vi "experiment control.vi"() -> ()   [LabVIEW 2012] (continued)
            n2214 = Decimal String To Number(string=w4963) -> (number=w4964:i32)  [unwired: 2 in, 1 out]
            n2215 = local read "DAC Schedule"() -> (w4965:T6)
            n2216 = local read "DAC Tasks"() -> (w4966:T8)
            n2217 = call "DAC compile.vi"("DAC Tasks"=w4966, "DAC Schedule"=w4965, "index"=w4964) -> ("DAC"=w4962:cluster{"Time":dbl, "Voltage":dbl[]}[])  [unwired: 8 in]
            n2218 = for {
              tunnel: w4962 -> [w4976] mode=indexing
              tunnel: [w4975] -> w4961 mode=indexing
              tunnel: [w4974] -> w4958 mode=indexing
              n2219 = Unbundle By Name(w4976) -> ("Time"=w4975:dbl, "Voltage"=w4974:dbl[])
            }
            n2220 = Transpose 2D Array(2D array=w4958) -> (transposed array=w4959:dbl[][])
            n2221 = for {
              tunnel: w4959 -> [w4972] mode=indexing
              tunnel: w4961 -> [w4973]
              tunnel: [w4971] -> w4960 mode=indexing
              n2222 = Bundle(w4973, w4972) -> (w4971:cluster{dbl[], dbl[]})  [unwired: 1 in]
            }
            "DAC View" <- w4960
          }
          frame "DAC: Clear" {
            n2223 = Unbundle By Name(w4982) -> ("dac state"=w4984:T7)
            n2224 = Unbundle By Name(w4984) -> ("loaded"=w4985:bool)
            n2225 = call <vilib>:"Clear Errors.vi"("error in (no error)"=w4978) -> ("error out"=w4980:errorcluster)  [unwired: 6 in]
            n2226 = case shown="True" w4985 {
              tunnel: [w4991 w5000] -> w4979
              tunnel: w4980 -> [w4994 w5000]
              tunnel: w4984 -> [w4988 w4999]
              tunnel: [w4987 w4999] -> w4983
              frame True {
                n2227 = Unbundle By Name(w4988) -> ("output 1"=w4998:refnum<k21>, "clock 1"=w4997:refnum<k21>, "output 2"=w4989:refnum<k21>, "clock 2"=w4990:refnum<k21>)
                n2228 = call <vilib>:"DAQmx Clear Task.vi"("task in"=w4998, "error in"=w4994) -> ("error out"=w4995:errorcluster)  [unwired: 13 in]
                n2229 = call <vilib>:"DAQmx Clear Task.vi"("task in"=w4997, "error in"=w4995) -> ("error out"=w4992:errorcluster)  [unwired: 13 in]
                n2230 = call <vilib>:"DAQmx Clear Task.vi"("task in"=w4989, "error in"=w4992) -> ("error out"=w4993:errorcluster)  [unwired: 13 in]
                n2231 = Bundle By Name(cluster=w4988, "loaded"=FALSE) -> (w4987:T7)
                n2232 = call <vilib>:"DAQmx Clear Task.vi"("task in"=w4990, "error in"=w4993) -> ("error out"=w4991:errorcluster)  [unwired: 13 in]
              }
              frame False {
              }
            }
            n2233 = Merge Errors(w4979, w4978) -> (w4977:errorcluster)
            n2234 = Bundle By Name(cluster=w4982, "dac state"=w4983) -> (w4981:T52)
          }
          frame "----------- Depletion Agilent -----------" {
            # "Template Separator\n(You can make a copy of, or modify, this frame)"
          }
          frame "Depletion Agilent: Initialize" {
            w5004 = TRUE ("Enable Output  (T: Enable)")
            # "Use this as a template for any command that you might want to profile."
            n2235 = local read "Depletion Agilent"() -> (w5006:T14)
            n2236 = Unbundle By Name(w5006) -> ("USB"=w5010:refnum<visa-resource-name>)
            n2237 = call <instrlib>:"Initialize.vi"("Serial Configuration"=T50 {"Baud Rate"=9600, "Parity"=0, "Data Bits"=8, "Flow Control"=4}, "error in (no error)"=w5013, "VISA resource name"=w5010) -> ("error out"=w5008:errorcluster, "VISA resource name out"=w5007:refnum<visa-resource-name>)  [unwired: 7 in]
            n2238 = call <instrlib>:"Enable Output.vi"("error in (no error)"=w5008, "Enable Output  (T: Enable)"=w5004, "VISA resource name"=w5007) -> ("error out"=w5012:errorcluster)  [unwired: 7 in, 1 out]
            n2239 = Bundle By Name(cluster=w5006, "Output"=w5004) -> (w5005:T14)
            n2240 = local write "Depletion Agilent"(w5005) -> ()
          }
          frame "Depletion Agilent: Set" {
            w5043 = u16 0 items=["50 Ohms", "High Impedance", "User Defined"] ("Impedance (0: 50 Ohms)")
            # "Use this as a template for any command that you might want to profile."
            n2241 = local read "Depletion Agilent"() -> (w5016:T14)
            n2242 = Unbundle By Name(w5016) -> ("Channels"=w5023:T96, "Output Select"=w5024:bool, "Amplitude"=w5020:dbl, "Offset"=w5019:dbl, "USB"=w5025:refnum<visa-resource-name>)
            n2243 = Boolean To (0,1)(Boolean=w5024) -> (0, 1=w5042:i16)
            n2244 = Delete From Array(array=w5023, index=w5042) -> (deleted portion=w5041:T97)  [unwired: 1 in, 1 out]
            n2245 = Unbundle By Name(w5041) -> ("Trigger"=w5018:bool, "Phase"=w5017:dbl, "Frequency"=w5022:dbl, "Duty Cycle"=w5021:dbl)
            n2246 = call <instrlib>:"Configure Output Impedance.vi"("error in (no error)"=w5045, "Impedance (0: 50 Ohms)"=w5043, "VISA resource name"=w5025) -> ("error out"=w5031:errorcluster, "VISA resource name out"=w5029:refnum<visa-resource-name>)  [unwired: 7 in]
            n2247 = Boolean To (0,1)(Boolean=w5018) -> (0, 1=w5035:i16)
            n2248 = Format Into String(format string="%.;:FREQ %f;:VOLT %g;:VOLT:OFFS %g;:FUNC:SQU:DCYC %f" ("Frequency Command"), initial string="FUNC:SHAP SQU;:VOLT:UNIT VPP;" ("string (\"\")"), w5022, w5020, w5019, w5021) -> (resulting string=w5034:string)  [unwired: 1 in, 1 out]
            n2249 = VISA Write(VISA resource name=w5029, write buffer=w5034, error in (no error)=w5031) -> (VISA resource name out=w5028:refnum<visa-resource-name>, error out=w5030:errorcluster)  [unwired: 1 out]
            n2250 = Pick Line(multi-line string="BURS:MODE TRIG;\nBURS:MODE GAT;" ("f"), line index=w5035) -> (output string=w5038:string)  [unwired: 1 in]
            n2251 = Format Into String(format string="%.;:BURS:PHAS %f;", initial string=w5038, w5017) -> (resulting string=w5027:string)  [unwired: 1 in, 1 out]
            n2252 = case shown="True" w5018 {
              tunnel: w5027 -> [w5049 w5052]
              tunnel: [w5047 w5050] -> w5026
              frame False {
                n2253 = Concatenate Strings(w5049, ":BURS:NCYC 10;:TRIG:SOUR IMM;") -> (w5047:string)
              }
              frame True {
                n2254 = Concatenate Strings(w5052, ":TRIG:SOUR EXT;:BURS:NCYC INF;") -> (w5050:string)
              }
            }
            n2255 = Concatenate Strings(w5026, ":BURS:STAT ON;") -> (w5032:string)
            n2256 = VISA Write(VISA resource name=w5028, write buffer=w5032, error in (no error)=w5030) -> (error out=w5015:errorcluster)  [unwired: 2 out]
          }
          frame "Depletion Agilent: Output" {
            # "Use this as a template for any command that you might want to profile."
            n2257 = local read "Depletion Agilent"() -> (w5055:T14)
            n2258 = Unbundle By Name(w5055) -> ("USB"=w5054:refnum<visa-resource-name>, "Output"=w5053:bool)
            n2259 = call <instrlib>:"Enable Output.vi"("error in (no error)"=w5058, "Enable Output  (T: Enable)"=w5053, "VISA resource name"=w5054) -> ("error out"=w5057:errorcluster)  [unwired: 7 in, 1 out]
          }
          frame "Depletion Agilent: Close" {
            # "Use this as a template for any command that you might want to profile."
            n2260 = local read "Depletion Agilent"() -> (w5062:T14)
            n2261 = Unbundle By Name(w5062) -> ("USB"=w5061:refnum<visa-resource-name>)
            n2262 = call <instrlib>:"Close.vi"("error in (no error)"=w5064, "VISA resource name"=w5061) -> ("error out"=w5063:errorcluster)  [unwired: 9 in]
          }
          frame "-----------Chillax-----------" {
            # "Template Separator\n(You can make a copy of, or modify, this frame)"
          }
          frame "Chillax: Initialize" {
            # "Use this as a template for any command that you might want to profile."
            n2263 = local read "Chillax"() -> (w5104:T12)
            n2264 = Unbundle By Name(w5104) -> ("Chillax Voltage"=w5097:dbl, "Chillax"=w5107:refnum<visa-resource-name>, "Output"=w5069:bool)
            n2265 = call <instrlib>:"Initialize.vi"("error in (no error)"=w5109, "VISA resource name"=w5107) -> ("error out"=w5106:errorcluster, "VISA resource name out"=w5105:refnum<visa-resource-name>)  [unwired: 8 in]
            n2266 = local read "Chillax"() -> (w5100:T12)
            n2267 = call <instrlib>:"Enable Output.vi"("error in (no error)"=w5106, "Enable Output  (T: Enable)"=w5069, "VISA resource name"=w5105) -> ("error out"=w5102:errorcluster, "VISA resource name out"=w5103:refnum<visa-resource-name>)  [unwired: 7 in]
            n2268 = Bundle By Name(cluster=w5100, "Output"=w5069) -> (w5099:T12)
            n2269 = Negate(x=w5097) -> (-x=w5096:dbl)
            n2270 = call "ag33xxx - Select User Def Wfm.vi"("error in (no error)"=w5102, "User Def. Wfm Name"="CHILLAX", "VISA session"=w5103) -> ("error out"=w5091:errorcluster, "dup VISA session"=w5092:refnum<visa-resource-name>)  [unwired: 7 in]
            n2271 = Format Into String(format string=":VOLT:HIGH 0;:VOLT:LOW %g;", w5096) -> (resulting string=w5090:string)  [unwired: 2 in, 1 out]
            n2272 = local write "Chillax"(w5099) -> ()
            n2273 = Format Into String(format string=":BURS:STAT ON;:BURS:MODE TRIG;:BURS:NCYC 1;:BURS:PHAS 0;:TRIG:SOUR EXT;:PULS:PER %g;", initial string=w5090, 0.013 ("input 1")) -> (resulting string=w5094:string)  [unwired: 1 in, 1 out]
            n2274 = VISA Write(VISA resource name=w5092, write buffer=w5094, error in (no error)=w5091) -> (error out=w5074:errorcluster)  [unwired: 2 out]
            n2275 = local read "Chillax"() -> (w5075:T12)
            n2276 = Unbundle By Name(w5075) -> ("Chillax Voltage"=w5071:dbl, "Unchillax"=w5072:refnum<visa-resource-name>, "Output"=w5070:bool)
            n2277 = call <instrlib>:"Initialize.vi"("error in (no error)"=w5074, "VISA resource name"=w5072) -> ("error out"=w5076:errorcluster, "VISA resource name out"=w5077:refnum<visa-resource-name>)  [unwired: 8 in]
            n2278 = local read "Chillax"() -> (w5081:T12)
            n2279 = call <instrlib>:"Enable Output.vi"("error in (no error)"=w5076, "Enable Output  (T: Enable)"=w5070, "VISA resource name"=w5077) -> ("error out"=w5079:errorcluster, "VISA resource name out"=w5078:refnum<visa-resource-name>)  [unwired: 7 in]
            n2280 = Bundle By Name(cluster=w5081, "Output"=w5070) -> (w5082:T12)
            n2281 = call "ag33xxx - Select User Def Wfm.vi"("error in (no error)"=w5079, "User Def. Wfm Name"="UNCHILLAX", "VISA session"=w5078) -> ("error out"=w5088:errorcluster, "dup VISA session"=w5087:refnum<visa-resource-name>)  [unwired: 7 in]
            n2282 = Format Into String(format string=":VOLT:LOW 0;:VOLT:HIGH %g;", w5071) -> (resulting string=w5089:string)  [unwired: 2 in, 1 out]
            n2283 = local write "Chillax"(w5082) -> ()
            n2284 = Format Into String(format string=":BURS:STAT ON;:BURS:MODE TRIG;:BURS:NCYC 1;:BURS:PHAS 0;:TRIG:SOUR EXT;:PULS:PER %g;", initial string=w5089, 0.13 ("input 1")) -> (resulting string=w5085:string)  [unwired: 1 in, 1 out]
            n2285 = VISA Write(VISA resource name=w5087, write buffer=w5085, error in (no error)=w5088) -> (error out=w5073:errorcluster)  [unwired: 2 out]
          }
          frame "Chillax: Close" {
            # "Use this as a template for any command that you might want to profile."
            n2286 = local read "Chillax"() -> (w5116:T12)
            n2287 = Unbundle By Name(w5116) -> ("Unchillax"=w5113:refnum<visa-resource-name>, "Chillax"=w5115:refnum<visa-resource-name>)
            n2288 = call "ag33xxx - Close.vi"("error in (no error)"=w5114, "VISA session"=w5115) -> ("error out"=w5112:errorcluster)  [unwired: 9 in]
            n2289 = call "ag33xxx - Close.vi"("error in (no error)"=w5112, "VISA session"=w5113) -> ("error out"=w5111:errorcluster)  [unwired: 9 in]
          }
          frame "Chillax: Set Voltage" {
            # "Use this as a template for any command that you might want to profile."
            n2290 = local read "Chillax"() -> (w5130:T12)
            n2291 = Unbundle By Name(w5130) -> ("Chillax Voltage"=w5120:dbl, "Chillax"=w5127:refnum<visa-resource-name>, "Unchillax"=w5119:refnum<visa-resource-name>)
            n2292 = Negate(x=w5120) -> (-x=w5121:dbl)
            n2293 = Format Into String(format string=":VOLT:HIGH 0;:VOLT:LOW %g;" ("Amplitude Command"), w5121) -> (resulting string=w5126:string)  [unwired: 2 in, 1 out]
            n2294 = VISA Write(VISA resource name=w5127, write buffer=w5126, error in (no error)=w5129) -> (error out=w5124:errorcluster)  [unwired: 2 out]
            n2295 = Format Into String(format string=":VOLT:LOW 0;:VOLT:HIGH %g;" ("Amplitude Command"), w5120) -> (resulting string=w5125:string)  [unwired: 2 in, 1 out]
            n2296 = VISA Write(VISA resource name=w5119, write buffer=w5125, error in (no error)=w5124) -> (error out=w5123:errorcluster)  [unwired: 2 out]
          }
          frame "Chillax: Output" {
            # "Use this as a template for any command that you might want to profile."
            n2297 = local read "Chillax"() -> (w5139:T12)
            n2298 = Unbundle By Name(w5139) -> ("Unchillax"=w5136:refnum<visa-resource-name>, "Chillax"=w5138:refnum<visa-resource-name>, "Output"=w5133:bool)
            n2299 = call <instrlib>:"Enable Output.vi"("error in (no error)"=w5137, "Enable Output  (T: Enable)"=w5133, "VISA resource name"=w5138) -> ("error out"=w5135:errorcluster)  [unwired: 7 in, 1 out]
            n2300 = call <instrlib>:"Enable Output.vi"("error in (no error)"=w5135, "Enable Output  (T: Enable)"=w5133, "VISA resource name"=w5136) -> ("error out"=w5134:errorcluster)  [unwired: 7 in, 1 out]
          }
          frame "----------- Trap Agilent -----------" {
            # "Template Separator\n(You can make a copy of, or modify, this frame)"
          }
          frame "Trap Agilent: Initialize" {
            w5145 = TRUE ("Enable Output  (T: Enable)")
            # "Use this as a template for any command that you might want to profile."
            n2301 = local read "Trap Agilent"() -> (w5147:T13)
            n2302 = Unbundle By Name(w5147) -> ("USB"=w5151:refnum<visa-resource-name>)
            n2303 = call <instrlib>:"Initialize.vi"("Serial Configuration"=T50 {"Baud Rate"=9600, "Parity"=0, "Data Bits"=8, "Flow Control"=4}, "error in (no error)"=w5154, "VISA resource name"=w5151) -> ("error out"=w5149:errorcluster, "VISA resource name out"=w5148:refnum<visa-resource-name>)  [unwired: 7 in]
            n2304 = call <instrlib>:"Enable Output.vi"("error in (no error)"=w5149, "Enable Output  (T: Enable)"=w5145, "VISA resource name"=w5148) -> ("error out"=w5153:errorcluster)  [unwired: 7 in, 1 out]
            n2305 = Bundle By Name(cluster=w5147, "Output"=w5145) -> (w5146:T13)
            n2306 = local write "Trap Agilent"(w5146) -> ()
          }
          frame "Trap Agilent: Set" {
            w5157 = u16 1 items=["DC", "Sine", "Square", "Triangle", "Ramp", "Pulse", "Noise", "Sinc", "Negative Ramp", "Exponential Rise", "Exponential Fall", "Cardiac"] ("Waveform Function (1: Sine)")
            w5163 = u16 0 items=["Vpp", "Vrms", "dB"] ("Unit (0: Vpp)")
            w5166 = u16 1 items=["50 Ohms", "High Impedance", "User Defined"] ("Impedance (0: 50 Ohms)")
            w5169 = u16 1 items=["Triggered", "Gated"] ("Burst Mode (0: Triggered)")
            # "Use this as a template for any command that you might want to profile."
            n2307 = local read "Trap Agilent"() -> (w5172:T13)
            n2308 = Unbundle By Name(w5172) -> ("Phase"=w5171:dbl, "Frequency"=w5173:dbl, "USB"=w5156:refnum<visa-resource-name>, "Amplitude"=w5164:dbl)
            n2309 = Divide(x=w5164, y=1000.0) -> (x/y=w5160:dbl)
            n2310 = Multiply(x=1000.0, y=w5173) -> (x*y=w5159:dbl)
            n2311 = call <instrlib>:"Configure Burst.vi"("Burst Mode (0: Triggered)"=w5169, "error in (no error)"=w5177, "Burst Phase (0 deg)"=w5171, "Enable Burst (T: Enable)"=TRUE, "VISA resource name"=w5156) -> ("error out"=w5168:errorcluster, "VISA resource name out"=w5167:refnum<visa-resource-name>)  [unwired: 5 in]
            n2312 = call <instrlib>:"Configure Output Impedance.vi"("error in (no error)"=w5168, "Impedance (0: 50 Ohms)"=w5166, "VISA resource name"=w5167) -> ("error out"=w5161:errorcluster, "VISA resource name out"=w5162:refnum<visa-resource-name>)  [unwired: 7 in]
            n2313 = call <instrlib>:"Configure Standard Waveform.vi"("Unit (0: Vpp)"=w5163, "DC Offset (0.00 V)"=0.0, "Frequency (1000 Hz)"=w5159, "error in (no error)"=w5161, "Amplitude (1)"=w5160, "Waveform Function (1: Sine)"=w5157, "VISA resource name"=w5162) -> ("error out"=w5176:errorcluster)  [unwired: 3 in, 1 out]
          }
          frame "Trap Agilent: Output" {
            # "Use this as a template for any command that you might want to profile."
            n2314 = local read "Trap Agilent"() -> (w5181:T13)
            n2315 = Unbundle By Name(w5181) -> ("USB"=w5180:refnum<visa-resource-name>, "Output"=w5179:bool)
            n2316 = call <instrlib>:"Enable Output.vi"("error in (no error)"=w5184, "Enable Output  (T: Enable)"=w5179, "VISA resource name"=w5180) -> ("error out"=w5183:errorcluster)  [unwired: 7 in, 1 out]
          }
          frame "Trap Agilent: Close" {
            # "Use this as a template for any command that you might want to profile."
            n2317 = local read "Trap Agilent"() -> (w5188:T13)
            n2318 = Unbundle By Name(w5188) -> ("USB"=w5187:refnum<visa-resource-name>)
            n2319 = call <instrlib>:"Close.vi"("error in (no error)"=w5190, "VISA resource name"=w5187) -> ("error out"=w5189:errorcluster)  [unwired: 9 in]
          }
          frame "----------- USB DAQ -----------" {
            # "Template Separator\n(You can make a copy of, or modify, this frame)"
          }
          frame "USB DAQ: Initialize" {
            # "Use this as a template for any command that you might want to profile."
            n2320 = local read "USB DAQ"() -> (w5208:T11)
            n2321 = Unbundle By Name(w5208) -> ("Analog Out"=w5202:u8[], "Digital Out"=w5197:bool[])
            n2322 = dll-call lib="C:/Users/edm/Desktop/experimentcontrol/trunk/subvis/USB DAQ/K8055D.dll" fn="OpenDevice"(error in=w5212, 0) -> (error out=w5209:errorcluster)  [unwired: 4 in, 1 out]
            n2323 = Not(x=w5197) -> (.not. x?=w5196:bool[])
            n2324 = Boolean Array To Number(Boolean array=w5196) -> (number=w5207:u32)
            n2325 = dll-call lib="C:/Users/edm/Desktop/experimentcontrol/trunk/subvis/USB DAQ/K8055D.dll" fn="WriteAllDigital"(error in=w5209, w5207) -> (error out=w5206:errorcluster)  [unwired: 4 in, 1 out]
            n2326 = Delete From Array(array=w5202, index=0) -> (deleted portion=w5201:u8)  [unwired: 1 in, 1 out]
            n2327 = dll-call lib="C:/Users/edm/Desktop/experimentcontrol/trunk/subvis/USB DAQ/K8055D.dll" fn="OutputAnalogChannel"(error in=w5206, 1, w5201) -> (error out=w5203:errorcluster)  [unwired: 5 in, 1 out]
            n2328 = Delete From Array(array=w5202, index=1) -> (deleted portion=w5200:u8)  [unwired: 1 in, 1 out]
            n2329 = dll-call lib="C:/Users/edm/Desktop/experimentcontrol/trunk/subvis/USB DAQ/K8055D.dll" fn="OutputAnalogChannel"(error in=w5203, 2, w5200) -> (error out=w5211:errorcluster)  [unwired: 5 in, 1 out]
          }
          frame "USB DAQ: Digital Write" {
            # "Use this as a template for any command that you might want to profile."
            n2330 = local read "USB DAQ"() -> (w5222:T11)
            n2331 = Match Pattern(string=w5232, regular expression=",") -> (before substring=w5228:string, after substring=w5227:string)  [unwired: 1 in, 2 out]
            n2332 = Decimal String To Number(string=w5227) -> (number=w5226:i32)  [unwired: 2 in, 1 out]
            n2333 = Unbundle By Name(w5222) -> ("Digital Out"=w5221:bool[])
            n2334 = Decimal String To Number(string=w5228) -> (number=w5225:i32)  [unwired: 2 in, 1 out]
            n2335 = Number To Boolean Array(number=w5226) -> (Boolean array=w5217:bool[])
            n2336 = Decrement(x=w5225) -> (x-1=w5224:i32)
            n2337 = Not(x=w5217) -> (.not. x?=w5216:bool[])
            n2338 = Not(x=w5221) -> (.not. x?=w5220:bool[])
            n2339 = Index Array(array=w5216, index=0) -> (element=w5214:bool)
            n2340 = Replace Array Subset(array=w5220, new element=w5214, index=w5224) -> (w5219:bool[])
            n2341 = Boolean Array To Number(Boolean array=w5219) -> (number=w5230:u32)
            n2342 = dll-call lib="C:/Users/edm/Desktop/experimentcontrol/trunk/subvis/USB DAQ/K8055D.dll" fn="WriteAllDigital"(error in=w5234, w5230) -> (error out=w5233:errorcluster)  [unwired: 4 in, 1 out]
            n2343 = Not(x=w5219) -> (.not. x?=w5218:bool[])
            n2344 = Bundle By Name(cluster=w5222, "Digital Out"=w5218) -> (w5223:T11)
            n2345 = local write "USB DAQ"(w5223) -> ()
          }
          frame "USB DAQ: Digital Read" {
            # "Use this as a template for any command that you might want to profile."
            n2346 = dll-call lib="C:/Users/edm/Desktop/experimentcontrol/trunk/subvis/USB DAQ/K8055D.dll" fn="ReadAllDigital"(error in=w5243) -> (error out=w5242:errorcluster, w5240:i32)  [unwired: 2 in, 1 out]
            n2347 = Number To Boolean Array(number=w5240) -> (Boolean array=w5237:bool[])
            n2348 = local read "USB DAQ"() -> (w5239:T11)
            n2349 = Not(x=w5237) -> (.not. x?=w5236:bool[])
            n2350 = Bundle By Name(cluster=w5239, "Digital In"=w5236) -> (w5238:T11)
            n2351 = local write "USB DAQ"(w5238) -> ()
          }
          frame "USB DAQ: Analog Write" {
            # "Use this as a template for any command that you might want to profile."
            n2352 = local read "USB DAQ"() -> (w5253:T11)
            n2353 = Unbundle By Name(w5253) -> ("Analog Out"=w5245:u8[])
            n2354 = Delete From Array(array=w5245, index=0) -> (deleted portion=w5252:u8)  [unwired: 1 in, 1 out]
            n2355 = dll-call lib="C:/Users/edm/Desktop/experimentcontrol/trunk/subvis/USB DAQ/K8055D.dll" fn="OutputAnalogChannel"(error in=w5256, 1, w5252) -> (error out=w5246:errorcluster)  [unwired: 5 in, 1 out]
            n2356 = Delete From Array(array=w5245, index=1) -> (deleted portion=w5247:u8)  [unwired: 1 in, 1 out]
            n2357 = dll-call lib="C:/Users/edm/Desktop/experimentcontrol/trunk/subvis/USB DAQ/K8055D.dll" fn="OutputAnalogChannel"(error in=w5246, 2, w5247) -> (error out=w5255:errorcluster)  [unwired: 5 in, 1 out]
          }
          frame "USB DAQ: Analog Read" {
            # "Use this as a template for any command that you might want to profile."
            n2358 = dll-call lib="C:/Users/edm/Desktop/experimentcontrol/trunk/subvis/USB DAQ/K8055D.dll" fn="ReadAllAnalog"(error in=w5265) -> (error out=w5264:errorcluster, w5261:i32, w5260:i32)  [unwired: 5 in, 1 out]
            n2359 = Build Array(w5261, w5260) -> (w5259:i32[])
            n2360 = local read "USB DAQ"() -> (w5263:T11)
            n2361 = Bundle By Name(cluster=w5263, "Analog In"=w5259) -> (w5262:T11)
            n2362 = local write "USB DAQ"(w5262) -> ()
          }
          frame "---------- QuadDVM ----------" {
            # "Template Separator\n(You can make a copy of, or modify, this frame)"
          }
          frame "QuadDVM: Initialize" {
            # "Use this as a template for any command that you might want to profile."
            n2363 = local read "QuadDVM"() -> (w5272:T31)
            n2364 = Unbundle By Name(w5272) -> ("Serial Port"=w5273:refnum<visa-resource-name>)
            n2365 = call-poly "VISA Configure Serial Port"("VISA resource name"=w5273, "timeout (10sec)"=u32 1000, "Enable Termination\nChar (T)"=FALSE ("Enable Termination\nChar (T)"), "baud rate (9600)"=u32 9600, "error in (no error)"=w5275) -> ("VISA resource name out"=w5281:refnum<visa-resource-name>, "error out"=w5280:errorcluster)  [unwired: 9 in]
            n2366 = VISA Write(VISA resource name=w5281, write buffer="FLSH 4\r" ("string"), error in (no error)=w5280) -> (VISA resource name out=w5271:refnum<visa-resource-name>, error out=w5274:errorcluster)  [unwired: 1 out]
            n2367 = Bundle By Name(cluster=w5272, "Serial Port"=w5271) -> (w5270:T31)
            n2368 = local write "QuadDVM"(w5270) -> ()
          }
          frame "QuadDVM: Read" {
            # "Use this as a template for any command that you might want to profile."
            n2369 = local read "QuadDVM"() -> (w5304:T31)
            n2370 = Unbundle By Name(w5304) -> ("Serial Port"=w5288:refnum<visa-resource-name>)
            n2371 = VISA Write(VISA resource name=w5288, write buffer="SNDT 4,\"VOLT? 0\"\r" ("string"), error in (no error)=w5293) -> (VISA resource name out=w5298:refnum<visa-resource-name>, error out=w5285:errorcluster)  [unwired: 1 out]
            n2372 = VISA Write(VISA resource name=w5298, write buffer="RAWN? 4,45\r" ("string"), error in (no error)=w5285) -> (VISA resource name out=w5296:refnum<visa-resource-name>, error out=w5297:errorcluster)  [unwired: 1 out]
            n2373 = VISA Read(VISA resource name=w5296, byte count=u32 45, error in (no error)=w5297) -> (read buffer=w5291:string, error out=w5292:errorcluster)  [unwired: 2 out]
            n2374 = Spreadsheet String To Array(delimiter (Tab)=",", format string="%f", spreadsheet string=w5291, array type (2D Dbl)=dbl[][] []) -> (array=w5301:dbl[][])
            n2375 = Reshape Array(w5301, 4 ("dimension size"), 1 ("dimension size")) -> (w5287:dbl[][])
            n2376 = Bundle By Name(cluster=w5304, "Quad DVM"=w5287) -> (w5303:T31)
            n2377 = local write "QuadDVM"(w5303) -> ()
          }
          frame "QuadDVM: Close" {
            # "Use this as a template for any command that you might want to profile."
            n2378 = local read "QuadDVM"() -> (w5307:T31)
            n2379 = Unbundle By Name(w5307) -> ("Serial Port"=w5306:refnum<visa-resource-name>)
            n2380 = VISA Close(VISA resource name=w5306, error in (no error)=w5310) -> (error out=w5309:errorcluster)
          }
          frame " ------- Temperature Monitor -------" {
            # "Template Separator\n(You can make a copy of, or modify, this frame)"
          }
          frame "Temperature: Read" {
            # "Use this as a template for any command that you might want to profile."
            n2381 = local read "Temperature Monitor"() -> (w5323:T29)
            n2382 = Unbundle By Name(w5323) -> ("last measurement time"=w5321:string)
            n2383 = Scan From String(format string="%<%Y-%m-%d %I:%M:%S %p >T", input string=w5321, error in=w5325) -> (error out=w5315:errorcluster, output 1=w5319:timestamp)  [unwired: 2 in, 2 out]
            n2384 = Get Date/Time In Seconds() -> (seconds since 1Jan1904=w5320:timestamp)
            n2385 = Subtract(x=w5320, y=w5319) -> (x-y=w5318:dbl)
            n2386 = Greater?(x=w5318, y=10.0) -> (0:w5316:bool)
            n2387 = case shown="True" w5316 {
              tunnel: w5315 -> [w5328 w5332]
              tunnel: [w5328 w5331] -> w5326
              tunnel: w5323 -> [_ w5329]
              frame False {
              }
              frame True {
                n2388 = call "temperature_monitor.vi"("error in"=w5332, "Temperature Monitor"=w5329) -> ("error out"=w5331:errorcluster, "Temperature Monitor"=w5330:T29)  [unwired: 8 in]
                n2389 = local write "Temperature Monitor"(w5330) -> ()
              }
            }
          }
          frame " ------- Magnetometer -------" {
            # "Template Separator\n(You can make a copy of, or modify, this frame)"
          }
          frame "Magnetometer: Initialize" {
            # "Use this as a template for any command that you might want to profile."
            n2390 = flat-sequence {
              tunnel: w5337 -> [w5342]
              tunnel: [w5341] -> w5336
              tunnel: w5336 -> [w5350]
              tunnel: [w5349] -> w5338
              frame #0 {
                n2391 = local read "Magnetometer"() -> (w5343:T28)
                n2392 = Unbundle By Name(w5343) -> ("USB ports"=w5344:refnum<visa-resource-name>[])
                n2393 = call "ConstellationClose.vi"("error in"=w5342, "Task out"=w5344) -> ("error out"=w5341:errorcluster)  [unwired: 9 in]
              }
              frame #1 {
                n2394 = local read "Magnetometer"() -> (w5354:T28)
                n2395 = Unbundle By Name(w5354) -> ("USB ports"=w5352:refnum<visa-resource-name>[], "Active Controllers"=w5351:cluster{"Status":bool, "Number":dbl}[])
                n2396 = call "ConstellationInit.vi"("Error in"=w5350, "Active Controllers"=w5351, "USB Ports"=w5352) -> ("Error out"=w5349:errorcluster, "Active Boards out"=w5346:cluster{"Status":bool, "Board":string}[][], "Active Controllers out"=w5347:cluster{"Status":bool, "Number":dbl}[], "Task out"=w5348:refnum<visa-resource-name>[])  [unwired: 5 in]
                n2397 = Bundle By Name(cluster=w5354, "USB ports"=w5348, "Active Controllers"=w5347, "Active Boards"=w5346, "Measurements"=T51 []) -> (w5353:T28)
                n2398 = local write "Magnetometer"(w5353) -> ()
              }
            }
          }
          frame "Magnetometer: Read" {
            # "Use this as a template for any command that you might want to profile."
            n2399 = local read "Magnetometer"() -> (w5359:T28)
            n2400 = Unbundle By Name(w5359) -> ("USB ports"=w5361:refnum<visa-resource-name>[], "Active Controllers"=w5360:cluster{"Status":bool, "Number":dbl}[], "Active Boards"=w5355:cluster{"Status":bool, "Board":string}[][])
            n2401 = call "ConstellationRead.vi"("error in"=w5363, "Active Boards"=w5355, "Active Controllers"=w5360, "Task in"=w5361) -> ("error out"=w5362:errorcluster, "Measurements"=w5356:T114, "Task out"=w5357:refnum<visa-resource-name>[])  [unwired: 5 in]
            n2402 = Bundle By Name(cluster=w5359, "USB ports"=w5357, "Measurements"=w5356) -> (w5358:T28)
            n2403 = local write "Magnetometer"(w5358) -> ()
          }
          frame "Magnetometer: Close" {
            # "Use this as a template for any command that you might want to profile."
            n2404 = local read "Magnetometer"() -> (w5367:T28)
            n2405 = Unbundle By Name(w5367) -> ("USB ports"=w5366:refnum<visa-resource-name>[])
            n2406 = call "ConstellationClose.vi"("error in"=w5369, "Task out"=w5366) -> ("error out"=w5368:errorcluster)  [unwired: 9 in]
          }
          frame "---------- Counter ----------" {
            # "Template Separator\n(You can make a copy of, or modify, this frame)"
          }
          frame "Counter: Initialize" {
            w5377 = u16 2 items=["duty cycle 1", "fall time 1", "frequency 1", "frequency 2", "frequency 3", "frequency ratio 1,2", "frequency ratio 1,3", "maximum 1", "maximum 2", "minimum 1", "minimum 2", "neg. pulse width 1", "period 1", "period 2", "period 3", "phase 1,2", "peak to peak 1", "peak to peak 2", "pos. pulse width 1", "rise time 1", "time interval 1,2", "*totalize continuous 1", "totalize timed 1"] ("function (2:frequency 1)")
            w5378 = u16 0 items=["configure", "measure?", "read?", "fetch?"] ("instruction (1:measure?)")
            # "Use this as a template for any command that you might want to profile."
            n2407 = local read "Frequency Counter"() -> (w5385:T30)
            n2408 = Unbundle By Name(w5385) -> ("GPIB Port"=w5386:refnum<visa-resource-name>)
            n2409 = call "HP53132A Initialize.vi"("error in (no error)"=w5388, "Reset (T: Reset)"=FALSE, "VISA resource"=w5386) -> ("error out"=w5382:errorcluster, "VISA session"=w5383:refnum<visa-resource-name>)  [unwired: 7 in]
            n2410 = disable-structure shown="Enabled" {
              disable-tunnel: w5383 -> [w5403 w5405]
              disable-tunnel: w5382 -> [w5402 w5404]
              disable-tunnel: [w5391 w5405] -> w5381
              disable-tunnel: [w5390 w5404] -> w5379
              frame Disabled {
                w5396 = u16 2 items=["Sensitivity: low", "Sensitivity: med", "Sensitivity: hi"] ("Sensitivity")
                w5401 = u16 2 items=["Sensitivity: low", "Sensitivity: med", "Sensitivity: hi"] ("Sensitivity")
                n2411 = call "HP 53132A Config Channels.vi"("VISA session"=w5403, "channel"=FALSE, "Sensitivity"=w5401, "error in (no error)"=w5402, "impedance"=TRUE, "attenuation"=FALSE) -> ("dup VISA session"=w5393:refnum<visa-resource-name>, "error out"=w5392:errorcluster)  [unwired: 12 in]
                n2412 = call "HP 53132A Config Channels.vi"("VISA session"=w5393, "channel"=TRUE, "Sensitivity"=w5396, "error in (no error)"=w5392, "impedance"=TRUE, "attenuation"=FALSE) -> ("dup VISA session"=w5391:refnum<visa-resource-name>, "error out"=w5390:errorcluster)  [unwired: 12 in]
              }
              frame Enabled {
              }
            }
            n2413 = call "HP 53132A Read a measurement.vi"("error in"=w5379, "function (2:frequency 1)"=w5377, "instruction (1:measure?)"=w5378, "VISA session"=w5381) -> ("error out"=w5387:T115, "dup VISA session"=w5380:refnum<visa-resource-name>)  [unwired: 1 in, 1 out]
            n2414 = Bundle By Name(cluster=w5385, "GPIB Port"=w5380) -> (w5384:T30)
            n2415 = local write "Frequency Counter"(w5384) -> ()
          }
          frame "Counter: Read" {
            # "Use this as a template for any command that you might want to profile."
            n2416 = local read "Frequency Counter"() -> (w5412:T30)
            n2417 = Unbundle By Name(w5412) -> ("GPIB Port"=w5410:refnum<visa-resource-name>, "Frequency"=w5408:dbl[])
            n2418 = case shown="\"1\", Default" w5413 {
              tunnel: w5410 -> [w5426 w5436 w5446]
              tunnel: [w5425 w5435 w5445] -> w5409
              tunnel: [w5424 w5434 w5444] -> w5414
              tunnel: w5415 -> [w5423 w5433 w5443]
              tunnel: w5408 -> [w5420 w5430 w5440]
              tunnel: [w5419 w5429 w5439] -> w5407
              frame "1", Default {
                w5421 = u16 2 items=["duty cycle 1", "fall time 1", "frequency 1", "frequency 2", "frequency 3", "frequency ratio 1,2", "frequency ratio 1,3", "maximum 1", "maximum 2", "minimum 1", "minimum 2", "neg. pulse width 1", "period 1", "period 2", "period 3", "phase 1,2", "peak to peak 1", "peak to peak 2", "pos. pulse width 1", "rise time 1", "time interval 1,2", "*totalize continuous 1", "totalize timed 1"] ("function (2:frequency 1)")
                w5422 = u16 3 items=["configure", "measure?", "read?", "fetch?"] ("instruction (1:measure?)")
                n2419 = call "HP 53132A Read a measurement.vi"("error in"=w5423, "function (2:frequency 1)"=w5421, "instruction (1:measure?)"=w5422, "VISA session"=w5426) -> ("error out"=w5424:T115, "Result"=w5417:dbl, "dup VISA session"=w5425:refnum<visa-resource-name>)  [unwired: 1 in]
                n2420 = Replace Array Subset(array=w5420, new element=w5417, index=0 ("index (row)")) -> (w5419:dbl[])
              }
              frame "2" {
                w5431 = u16 3 items=["duty cycle 1", "fall time 1", "frequency 1", "frequency 2", "frequency 3", "frequency ratio 1,2", "frequency ratio 1,3", "maximum 1", "maximum 2", "minimum 1", "minimum 2", "neg. pulse width 1", "period 1", "period 2", "period 3", "phase 1,2", "peak to peak 1", "peak to peak 2", "pos. pulse width 1", "rise time 1", "time interval 1,2", "*totalize continuous 1", "totalize timed 1"] ("function (2:frequency 1)")
                w5432 = u16 2 items=["configure", "measure?", "read?", "fetch?"] ("instruction (1:measure?)")
                n2421 = call "HP 53132A Read a measurement.vi"("error in"=w5433, "function (2:frequency 1)"=w5431, "instruction (1:measure?)"=w5432, "VISA session"=w5436) -> ("error out"=w5434:T115, "Result"=w5427:dbl, "dup VISA session"=w5435:refnum<visa-resource-name>)  [unwired: 1 in]
                n2422 = Replace Array Subset(array=w5430, new element=w5427, index=1 ("index (row)")) -> (w5429:dbl[])
              }
              frame "3" {
                w5441 = u16 4 items=["duty cycle 1", "fall time 1", "frequency 1", "frequency 2", "frequency 3", "frequency ratio 1,2", "frequency ratio 1,3", "maximum 1", "maximum 2", "minimum 1", "minimum 2", "neg. pulse width 1", "period 1", "period 2", "period 3", "phase 1,2", "peak to peak 1", "peak to peak 2", "pos. pulse width 1", "rise time 1", "time interval 1,2", "*totalize continuous 1", "totalize timed 1"] ("function (2:frequency 1)")
                w5442 = u16 2 items=["configure", "measure?", "read?", "fetch?"] ("instruction (1:measure?)")
                n2423 = call "HP 53132A Read a measurement.vi"("error in"=w5443, "function (2:frequency 1)"=w5441, "instruction (1:measure?)"=w5442, "VISA session"=w5446) -> ("error out"=w5444:T115, "Result"=w5437:dbl, "dup VISA session"=w5445:refnum<visa-resource-name>)  [unwired: 1 in]
                n2424 = Replace Array Subset(array=w5440, new element=w5437, index=2 ("index (row)")) -> (w5439:dbl[])
              }
            }
            n2425 = Bundle By Name(cluster=w5412, "GPIB Port"=w5409, "Frequency"=w5407) -> (w5411:T30)
            n2426 = local write "Frequency Counter"(w5411) -> ()
          }
          frame "Counter: Close" {
            # "Use this as a template for any command that you might want to profile."
            n2427 = local read "Frequency Counter"() -> (w5448:T30)
            n2428 = Unbundle By Name(w5448) -> ("GPIB Port"=w5447:refnum<visa-resource-name>)
            n2429 = VISA Close(VISA resource name=w5447, error in (no error)=w5451) -> (error out=w5450:errorcluster)
          }
          frame "---------- Microwave ----------" {
            # "Template Separator\n(You can make a copy of, or modify, this frame)"
          }
          frame "Microwave: Setup" {
            # "Use this as a template for any command that you might want to profile."
            n2430 = while {
              shift-right: [w5472] -> _
              shift-left: "Microwave: RF\nMicrowave: Pulse\nMicrowave: Set Frequency\nMicrowave: Pulse\nMicrowave: Set Sweep Time\nMicrowave: Set Sweep" -> [w5474]
              tunnel: [w5471] -> w5462 mode=indexing
              stop <- w5469 stop-if-true
              n2431 = Match Pattern(string=w5474, regular expression="[\\n\\r]+") -> (before substring=w5471:string, after substring=w5472:string, offset past match=w5470:i32)  [unwired: 1 in, 1 out]
              n2432 = Less Than 0?(x=w5470) -> (x < 0?=w5469:bool)
            }
            n2433 = Reverse 1D Array(array=w5462) -> (reversed array=w5461:string[])
            n2434 = for {
              tunnel: [w5468] -> w5458
              tunnel: w5459 -> [w5467]
              shift-right: [w5465] -> w5456
              shift-left: w5457 -> [w5466]
              tunnel: w5461 -> [w5464] mode=indexing
              n2435 = Enqueue Element At Opposite End(queue=w5467, element=w5464, error in (no error)=w5466) -> (queue out=w5468:refnum<queue>, error out=w5465:errorcluster)  [unwired: 1 in, 1 out]
            }
          }
          frame "Microwave: RF" {
            # "Use this as a template for any command that you might want to profile."
            n2436 = local read "HP8341B"() -> (w5477:T27)
            n2437 = Unbundle By Name(w5477) -> ("detected"=w5476:bool)
            n2438 = case shown="True" w5476 {
              tunnel: w5477 -> [_ w5492]
              tunnel: [w5481 w5490] -> w5478
              tunnel: w5479 -> [w5481 w5489]
              frame False {
              }
              frame True {
                n2439 = Unbundle By Name(w5492) -> ("GPIB Port"=w5488:refnum<visa-resource-name>, "rf"=w5482:bool)
                n2440 = Boolean To (0,1)(Boolean=w5482) -> (0, 1=w5483:i16)
                n2441 = Number To Fractional String(number=w5483) -> (F-format string=w5486:string)  [unwired: 3 in]
                n2442 = Concatenate Strings("RF" ("string"), w5486) -> (w5484:string)
                n2443 = VISA Write(VISA resource name=w5488, write buffer=w5484, error in (no error)=w5489) -> (VISA resource name out=w5487:refnum<visa-resource-name>, error out=w5490:errorcluster)  [unwired: 1 out]
                n2444 = Bundle By Name(cluster=w5492, "GPIB Port"=w5487) -> (w5491:T27)
                n2445 = local write "HP8341B"(w5491) -> ()
              }
            }
          }
          frame "Microwave: Pulse" {
            # "Use this as a template for any command that you might want to profile."
            n2446 = local read "HP8341B"() -> (w5495:T27)
            n2447 = Unbundle By Name(w5495) -> ("detected"=w5494:bool)
            n2448 = case shown="True" w5494 {
              tunnel: w5495 -> [_ w5510]
              tunnel: [w5499 w5508] -> w5496
              tunnel: w5497 -> [w5499 w5507]
              frame False {
              }
              frame True {
                n2449 = Unbundle By Name(w5510) -> ("GPIB Port"=w5506:refnum<visa-resource-name>, "Pulse Modulate"=w5500:bool)
                n2450 = Boolean To (0,1)(Boolean=w5500) -> (0, 1=w5501:i16)
                n2451 = Number To Fractional String(number=w5501) -> (F-format string=w5504:string)  [unwired: 3 in]
                n2452 = Concatenate Strings("PM" ("string"), w5504) -> (w5502:string)
                n2453 = VISA Write(VISA resource name=w5506, write buffer=w5502, error in (no error)=w5507) -> (VISA resource name out=w5505:refnum<visa-resource-name>, error out=w5508:errorcluster)  [unwired: 1 out]
                n2454 = Bundle By Name(cluster=w5510, "GPIB Port"=w5505) -> (w5509:T27)
                n2455 = local write "HP8341B"(w5509) -> ()
              }
            }
          }
          frame "Microwave: Set Frequency" {
            # "Use this as a template for any command that you might want to profile."
            n2456 = local read "HP8341B"() -> (w5513:T27)
            n2457 = Unbundle By Name(w5513) -> ("detected"=w5512:bool)
            n2458 = case shown="True" w5512 {
              tunnel: w5513 -> [_ w5532]
              tunnel: [w5517 w5530] -> w5514
              tunnel: w5515 -> [w5517 w5529]
              frame False {
              }
              frame True {
                n2459 = Unbundle By Name(w5532) -> ("GPIB Port"=w5528:refnum<visa-resource-name>, "frequency"=w5520:dbl)
                n2460 = Add(x=w5520, y=35869.0) -> (x+y=w5519:dbl)
                n2461 = Divide(x=w5519, y=2.0) -> (x/y=w5518:dbl)
                n2462 = Number To Fractional String(number=w5518) -> (F-format string=w5526:string)  [unwired: 3 in]
                n2463 = Concatenate Strings("CW" ("string"), w5526, "MZ" ("string")) -> (w5523:string)
                n2464 = VISA Write(VISA resource name=w5528, write buffer=w5523, error in (no error)=w5529) -> (VISA resource name out=w5527:refnum<visa-resource-name>, error out=w5530:errorcluster)  [unwired: 1 out]
                n2465 = Bundle By Name(cluster=w5532, "GPIB Port"=w5527, "Set frequency"=w5518) -> (w5531:T27)
                n2466 = local write "HP8341B"(w5531) -> ()
              }
            }
          }
          frame "Microwave: Set Power" {
            # "Use this as a template for any command that you might want to profile."
            n2467 = local read "HP8341B"() -> (w5535:T27)
            n2468 = Unbundle By Name(w5535) -> ("detected"=w5534:bool)
            n2469 = case shown="True" w5534 {
              tunnel: w5535 -> [_ w5550]
              tunnel: [w5539 w5548] -> w5536
              tunnel: w5537 -> [w5539 w5547]
              frame False {
              }
              frame True {
                n2470 = Unbundle By Name(w5550) -> ("GPIB Port"=w5546:refnum<visa-resource-name>, "power"=w5544:dbl)
                n2471 = Number To Fractional String(number=w5544) -> (F-format string=w5543:string)  [unwired: 3 in]
                n2472 = Concatenate Strings("PL" ("string"), w5543, "DB" ("string")) -> (w5540:string)
                n2473 = VISA Write(VISA resource name=w5546, write buffer=w5540, error in (no error)=w5547) -> (VISA resource name out=w5545:refnum<visa-resource-name>, error out=w5548:errorcluster)  [unwired: 1 out]
                n2474 = Bundle By Name(cluster=w5550, "GPIB Port"=w5545) -> (w5549:T27)
                n2475 = local write "HP8341B"(w5549) -> ()
              }
            }
          }
          frame "Microwave: Set Sweep Time" {
            # "Use this as a template for any command that you might want to profile."
            n2476 = local read "HP8341B"() -> (w5552:T27)
            n2477 = Unbundle By Name(w5552) -> ("detected"=w5551:bool)
            n2478 = case shown="True" w5551 {
              tunnel: w5552 -> [_ w5568]
              tunnel: [w5557 w5566] -> w5554
              tunnel: w5555 -> [w5557 w5565]
              frame False {
              }
              frame True {
                n2479 = Unbundle By Name(w5568) -> ("GPIB Port"=w5564:refnum<visa-resource-name>, "sweep time"=w5562:dbl)
                n2480 = Number To Fractional String(number=w5562) -> (F-format string=w5561:string)  [unwired: 3 in]
